vi "Read Post AIV Values.vi"(8 "error in":errorcluster, 11 "DAC HeatFlow AIV in":refnum<class "DAC HeatFlow AIV.lvclass">) -> (0 "error out":errorcluster, 3 "DAC HeatFlow AIV out":refnum<class "DAC HeatFlow AIV.lvclass">)   [LabVIEW 2019, in "DAC.lvlib" / "DAC HeatFlow AIV.lvclass"]
uses:
  DAC HeatFlow AIV.lvclass
  Results/Results Method.ctl
  Results/Heat Flow Results/Heat Flow Results.lvclass
  DAC HeatFlow AIV.lvclass/DAC HeatFlow AIV.ctl
  <vilib>/DAQmx/read.llb/DAQmx Read (Analog Wfm 1Chan NSamp).vi
  <vilib>/Analysis/baseanly.llb/Mean (DBL).vi
  <vilib>/DAQmx/miscellaneous.llb/DAQmx Fill In Error Info.vi
  <vilib>/Analysis/NI_AALBase.lvlib
  Results/Results.lvlib
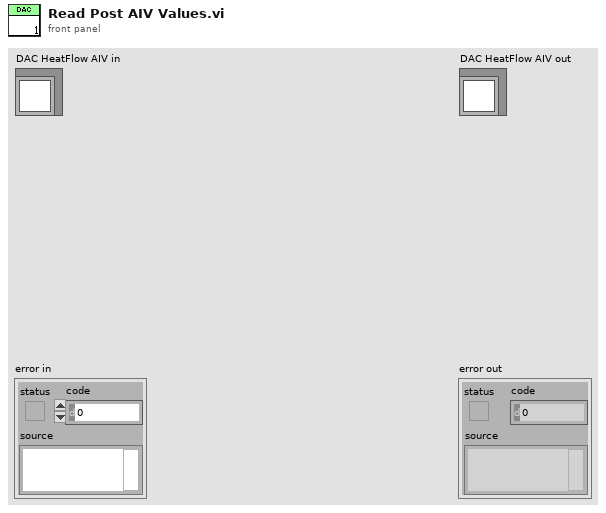
[diagram p1: front panel]
types:
  T1 = typedef "Results.lvlib/Results Method.ctl" = enum16{"Get", "Set"}
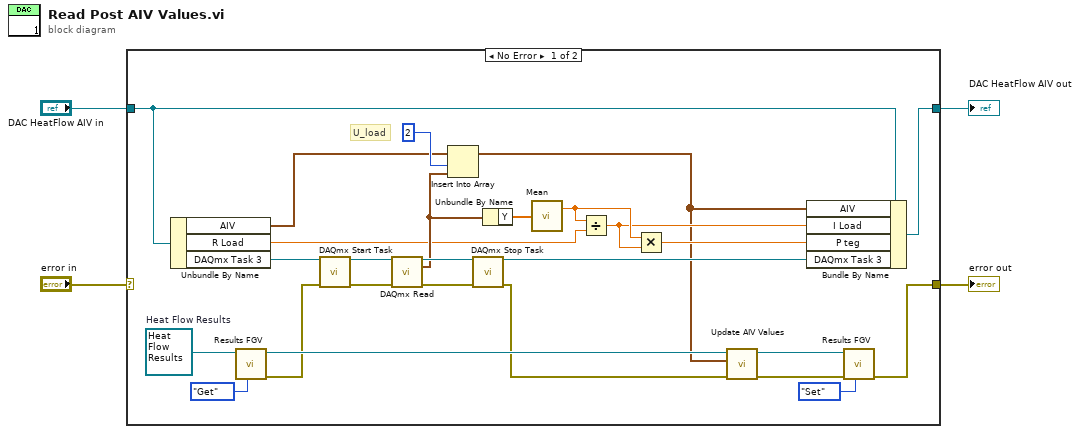
[diagram p0: block diagram]
diagram:
  n1 = case shown="No Error" "error in" {
    selector: "error in" -> [_ w32]
    tunnel: [w6 w32] -> w3
    tunnel: [w30 w31] -> w1
    tunnel: "DAC HeatFlow AIV in" -> [w29 w31]
    frame No Error {
      w12 = refnum<class "Heat Flow Results.lvclass"> refnum  # Heat Flow Results
      # "U_load"
      n2 = Unbundle By Name(w29) -> ("AIV"=w17:waveform(dbl)[], "R Load"=w16:dbl, "DAQmx Task 3"=w28:refnum<k21>)
      n3 = call-dynamic "Results FGV.vi"("Method"=Results_Method."Get", "Results in"=w12) -> ("error out"=w9:errorcluster, "Results out"=w11:refnum<class "Heat Flow Results.lvclass">)  [unwired: 8 in]
      n4 = call <vilib>:"DAQmx Start Task.vi"("task/channels in"=w28, "error in"=w9) -> ("task out"=w27:refnum<k21>, "error out"=w24:errorcluster)  [unwired: 12 in]
      n5 = call-poly <vilib>:"DAQmx Read.vi"("task/channels in"=w27, "error in"=w24) -> ("task out"=w26:refnum<k21>, "data"=w21:waveform(dbl), "error out"=w23:errorcluster)  [unwired: 11 in]
      n6 = Insert Into Array "Insert Into Array"(array=w17, index=2, new element=w21) -> (w5:waveform(dbl)[])
      n7 = call <vilib>:"DAQmx Stop Task.vi"("task/channels in"=w26, "error in"=w23) -> ("task out"=w25:refnum<k21>, "error out"=w8:errorcluster)  [unwired: 12 in]
      n8 = Unbundle By Name(w21) -> ("Y"=w20:dbl[])
      n9 = call-poly <vilib>:"Mean.vi"("X"=w20) -> ("mean"=w14:dbl)  [unwired: 1 out]
      n10 = Divide(x=w14, y=w16) -> (x/y=w13:dbl)
      n11 = Multiply(x=w14, y=w13) -> (x*y=w15:dbl)
      n12 = call "Update AIV Values.vi"("error in"=w8, "AIV"=w5, "Heat Flow Results in"=w11) -> ("error out"=w7:errorcluster, "Heat Flow Results out"=w10:refnum<class "Heat Flow Results.lvclass">)  [unwired: 7 in]
      n13 = Bundle By Name(cluster=w29, "AIV"=w5, "I Load"=w13, "P teg"=w15, "DAQmx Task 3"=w25) -> (w30:refnum<class "DAC HeatFlow AIV.lvclass">)
      n14 = call-dynamic "Results FGV.vi"("Method"=Results_Method."Set", "error in"=w7, "Results in"=w10) -> ("error out"=w6:errorcluster)  [unwired: 7 in, 1 out]
    }
    frame Error {
    }
  }
  "error out" <- w3
  "DAC HeatFlow AIV out" <- w1
